vi "NI VeriStand - Get Single Parameter Value.vi"(7 "Target":string, 8 "error in (no error)":errorcluster, 10 "Parameter":string, 11 "ModelManager in":T1) -> (0 "error out":errorcluster, 2 "Value":dbl, 3 "ModelManager out":T1)   [LabVIEW 2020, in "NI_VS ModelManager ExecutionAPI.lvlib"]
doc: "Returns values of model parameters present on the target. You must manually select the polymorphic instance to use."
uses:
  <vilib>/NI VeriStand/Execution/ModelManager/NI_VS ModelManager ExecutionAPI.lvlib
  <vilib>/NI VeriStand/Execution/ModelManager/ModelManagerAPI.ctl
  NationalInstruments.VeriStand.ClientAPI
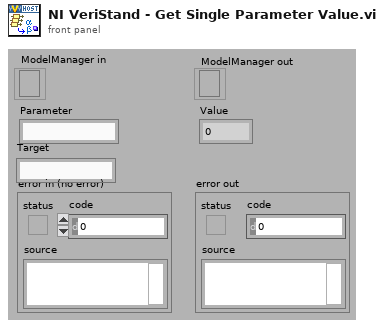
[diagram p1: front panel]
types:
  T1 = typedef "NI_VS ModelManager ExecutionAPI.lvlib/ModelManagerAPI.ctl" = refnum<k24>
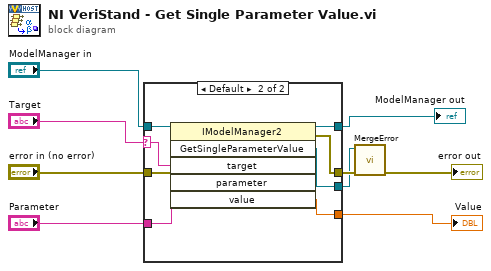
[diagram p0: block diagram]
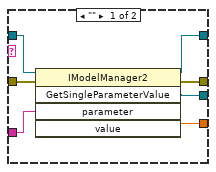
[diagram p2: hidden frame]
diagram:
  n1 = case shown="Default" "Target" {
    selector: "Target" -> [_ w18]
    tunnel: "ModelManager in" -> [w16 w24]
    tunnel: [w15 w23] -> w8
    tunnel: [w14 w22] -> w7
    tunnel: [w13 w21] -> w6
    tunnel: "error in (no error)" -> [w12 w20]
    tunnel: "Parameter" -> [w11 w19]
    tunnel: [w10 w17] -> w2
    frame "" {
      n2 = invoke class="IModelManager2" method="GetSingleParameterValue"(reference=w16, error in=w12, "parameter"=w11) -> (reference out=w15:T1, error out=w14:errorcluster, "GetSingleParameterValue"=w13:refnum<k24>, "value"=w10:dbl)  [unwired: 2 in, 1 out]
    }
    frame Default {
      n3 = invoke class="IModelManager2" method="GetSingleParameterValue"(reference=w24, error in=w20, "target"=w18, "parameter"=w19) -> (reference out=w23:T1, error out=w22:errorcluster, "GetSingleParameterValue"=w21:refnum<k24>, "value"=w17:dbl)  [unwired: 2 in, 2 out]
    }
  }
  "ModelManager out" <- w8
  "Value" <- w2
  n4 = call <vilib>:"MergeError.vi"("error in (no error)"=w7, "Error"=w6) -> ("error out"=→"error out":errorcluster)  [unwired: 9 out]
